vi "zad1.vi"() -> ()   [LabVIEW 2017]
uses:
  <vilib>/sound2/lvsound2.llb/Sound Data Format.ctl
  <vilib>/sound2/lvsound2.llb/Sampling Mode.ctl
  <vilib>/sound2/lvsound2.llb/Sound Input Read (DBL).vi
panel:
  out "Waveform Graph":waveform(dbl)[](graph)
  in  "stop":bool
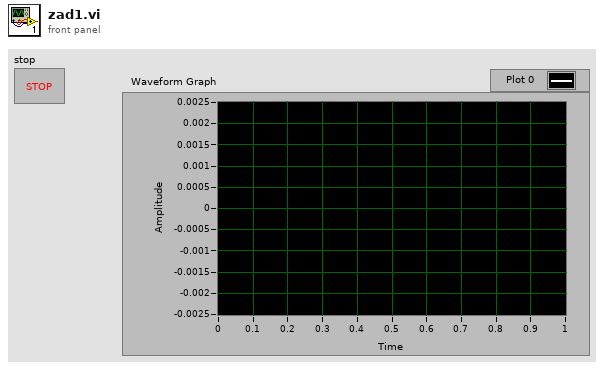
[diagram p1: front panel]
types:
  T1 = typedef "Sampling Mode.ctl" = i32
  T2 = typedef "Sound Data Format.ctl" = cluster{"sample rate (S/s)":dbl, "number of channels":i32, "bits per sample":i32}
  T3 = typedef "Sound Input Task ID.ctl" = u32
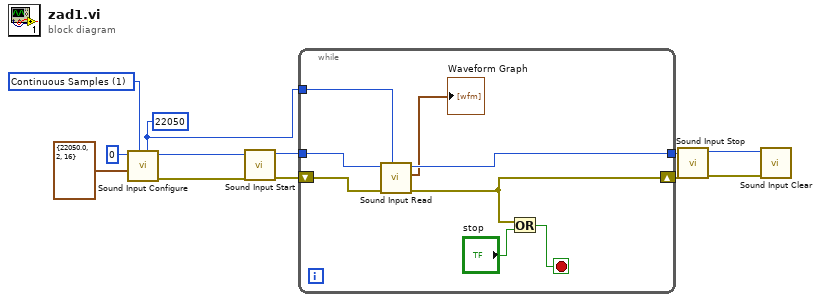
[diagram p0: block diagram]
diagram:
  w4 = T1 1 items=["Finite Samples", "Continuous Samples"] ("sample mode")
  w1 = 22050 ("number of samples/ch")
  n1 = call <vilib>:"Sound Input Configure.vi"("number of samples/ch"=w1, "sample mode"=w4, "sound format"=T2 {"sample rate (S/s)"=22050.0, "number of channels"=2, "bits per sample"=16}, "device ID"=u32 0) -> ("error out"=w11:errorcluster, "task ID"=w6:T3)  [unwired: 6 in]
  n2 = call <vilib>:"Sound Input Start.vi"("error in (no error)"=w11, "task ID"=w6) -> ("error out"=w10:errorcluster, "task ID out"=w5:T3)  [unwired: 8 in]
  n3 = while {
    tunnel: w5 -> [w19]
    tunnel: w1 -> [w18]
    shift-right: [w16] -> w9
    shift-left: w10 -> [w20]
    tunnel: [w14] -> w3
    stop <- w15 stop-if-true
    n4 = call-poly <vilib>:"Sound Input Read.vi"("number of samples/ch"=w18, "error in (no error)"=w20, "task ID"=w19) -> ("error out"=w16:errorcluster, "data"=→"Waveform Graph":waveform(dbl)[], "task ID out"=w14:T3)  [unwired: 6 in]
    n5 = Or(x=w16, y="stop") -> (x .or. y?=w15:bool)
  }
  n6 = call <vilib>:"Sound Input Stop.vi"("error in (no error)"=w9, "task ID"=w3) -> ("error out"=w8:errorcluster, "task ID out"=w2:T3)  [unwired: 8 in]
  n7 = call <vilib>:"Sound Input Clear.vi"("error in (no error)"=w8, "task ID"=w2) -> ()  [unwired: 9 in, 1 out]
